vi "AWS_DataFinder_DisplaySignal_Graph.vi"(8 "error in":errorcluster {"code" min=0 max=0}, 10 "result references":refnum<k20>[](array[refnum])) -> (0 "error out":errorcluster, 1 "slope":dbl, 2 "XY Graph":T1(graph))   [LabVIEW 2014]
doc: "Displays resulting signals as waveforms."
uses:
  <vilib>/DataFinder/DataTypes/property.ctl
  <vilib>/DataFinder/DataTypes/object type.ctl
  <vilib>/DataFinder/DataTypes/data type.ctl
  <vilib>/DataFinder/Get Property Values (Numeric Property).vi
  <vilib>/DataFinder/Get Property Values (Date Property).vi
  <vilib>/DataFinder/NI_DataFinder Toolkit.lvlib
  <vilib>/Analysis/NI_AALPro.lvlib
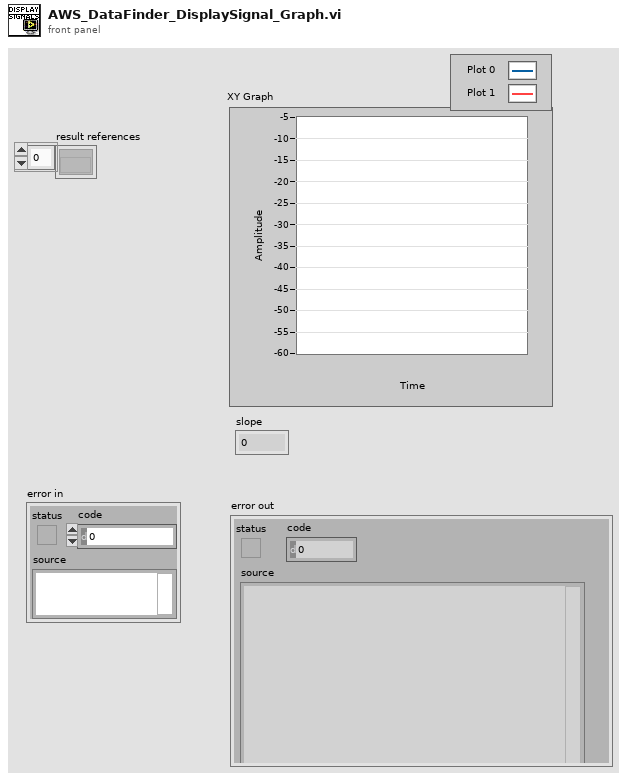
[diagram p1: front panel]
types:
  T1 = cluster{"property values":timestamp[], "Best Linear Fit":dbl[]}[]
  T2 = typedef "NI_DataFinder Toolkit.lvlib/property.ctl" = cluster{"object type":T3, "property name":string, "data type":T4}
  T3 = typedef "NI_DataFinder Toolkit.lvlib/object type.ctl" = u16
  T4 = typedef "NI_DataFinder Toolkit.lvlib/data type.ctl" = u16
  T5 = typedef "NI_DataFinder Controls.lvlib/DFSearchResult.ctl" = refnum<k20>
  T6 = cluster{"property values":timestamp[], "property values":dbl[]}
  T7 = cluster{"property values":timestamp[], "Best Linear Fit":dbl[]}
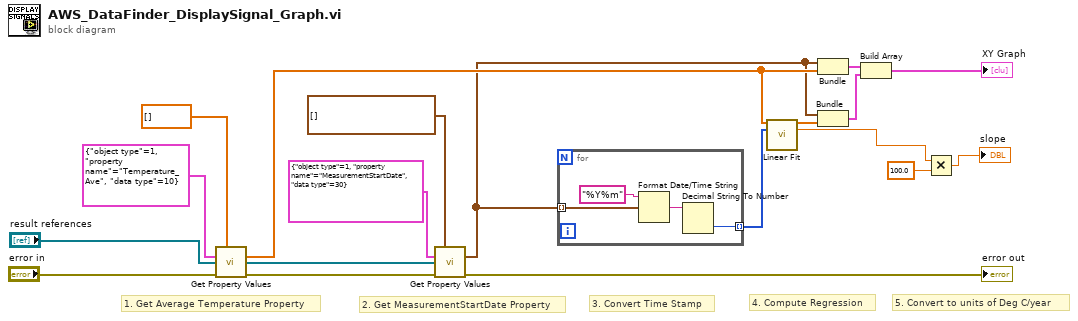
[diagram p0: block diagram]
diagram:
  # "4. Compute Regression"
  # "3. Convert Time Stamp"
  # "2. Get MeasurementStartDate Property"
  # "1. Get Average Temperature Property"
  # "5. Convert to units of Deg C/year"
  n1 = call-poly <vilib>:"Get Property Values.vi"("data type"=dbl[] [], "property"=T2 {"object type"=1, "property name"="Temperature_Ave", "data type"=10}, "result references"="result references", "error in (no error)"="error in") -> ("property values"=w10:dbl[], "result references out"=w13:T5[], "error out"=w12:errorcluster)  [unwired: 9 in]
  n2 = call-poly <vilib>:"Get Property Values.vi"("data type"=timestamp[] [] ("Timestamp"), "property"=T2 {"object type"=1, "property name"="MeasurementStartDate", "data type"=30}, "result references"=w13, "error in (no error)"=w12) -> ("property values"=w6:timestamp[], "error out"=→"error out":errorcluster)  [unwired: 9 in, 1 out]
  n3 = for {
    tunnel: [w21] -> w8 mode=indexing
    tunnel: w6 -> [w20] mode=indexing
    n4 = Format Date/Time String(time format string (%c)="%Y%m", seconds (now)=w20) -> (date/time string=w22:string)  [unwired: 1 in]
    n5 = Decimal String To Number(string=w22) -> (number=w21:i32)  [unwired: 2 in, 1 out]
  }
  n6 = call <vilib>:"Linear Fit.vi"("Y"=w10, "X"=w8) -> ("Best Linear Fit"=w9:dbl[], "slope"=w3:dbl)  [unwired: 9 in, 3 out]
  n7 = Bundle("property values"=w6, "property values"=w10) -> (w7:T6)  [unwired: 1 in]
  n8 = Bundle("property values"=w6, "Best Linear Fit"=w9) -> (w4:T7)  [unwired: 1 in]
  n9 = Build Array(w7, w4) -> (→"XY Graph":T1)
  n10 = Multiply(x=w3, y=100.0) -> (x*y=→"slope":dbl)
